vi "SV TDMS Write Even-Angle Channel Info.vi"(0 "tdms file":refnum<k34>, 1 "even-angle channel info":T6 {"channel info"."pregain" format="%.2f"; "channel info"."weighting filter" items=["Linear", "A-weighting", "B-weighting", "C-weighting", "ITU-R 468-4", "Dolby", "CCITT", "C-message", "Wb", "Wc", "Wd", "We", "Wf", "Wh", "Wj", "Wk", "Wm", "AES17 20 kHz lowpass", "AES17 40 kHz lowpass", "AES17 20 kHz highpass", "AES17 40 kHz highpass"]; "channel info"."dB reference" format="%^.1e"; "channel info"."engineering units" items=["custom..."=0, "V"=1, "A"=21, "C"=30, "pC"=31, "s"=32, "-"=29, "Pa"=2, "N"=20, "g"=3, "m/s^2"=4, "m/s"=5, "m"=6, "mm/s"=12, "mm"=13, "micron/s"=14, "micron"=15, "in/s^2"=7, "in/s"=8, "in"=9, "mil/s"=10, "mil"=11, "rad/s^2"=16, "rad/s"=17, "rad"=18, "deg/s^2"=26, "deg/s"=27, "deg"=28, "RPM"=22, "cycle/s^2"=23, "Hz"=24, "cycle"=25, "strain"=19]; "channel info"."sensor sensitivity" format="%#_5f"}, 5 "group name in":string, 7 "channel name in":string, 11 "error in":errorcluster) -> (4 "tdms file out":refnum<k34>, 6 "group name out":string, 8 "channel name out":string, 13 "function info":T5 {"function type" items=["Signal"=0, "Speed"=3, "Ratio"=6, "Count"=7, "-"=9, "Level"=10, "-"=19, "Octave Spectrum"=20, "-"=29, "FFT Auto Spectrum"=30, "FFT Cross Spectrum"=40, "Frequency Response"=50, "-"=59, "Event"=90]; "function subtype" items=["Unscaled binary"=0, "Scaled voltage"=1, "Scaled engineering units"=2, "-"=10, "Value"=19, "DC"=11, "AC"=12, "RMS^2"=13, "RMS"=14, "Peak"=15, "Peak to peak"=16, "-"=20, "1/1 octave"=21, "1/3 octave"=22, "1/6 octave"=23, "1/12 octave"=24, "1/24 octave"=25, "-"=30, "Density"=31, "Magnitude"=32, "Phase"=33, "Real"=34, "Imaginary"=35, "Complex"=345, "Coherence"=36, "-"=90, "Unknown"=99]; "X-domain" items=["Time (s)"=0, "Frequency-CB (Hz)"=1, "Frequency-CPB (Hz)"=1248, "Frequency-Arbitrary (Hz)"=2357, "Quefrency (s)"=2, "Revolutions (rev)"=3, "Order"=4, "Speed (RPM)"=11, "Speed (rad/s)"=21, "Index"=65535]}, 14 "unit info":T1, 15 "error out":errorcluster)   [LabVIEW 2017]
uses:
  <vilib>/addons/_NISVFA/_Shared subVIs/Controls/svc_Resampled Channel Info.ctl
  <vilib>/addons/_NISVFA/_Shared subVIs/Controls/svc_Channel Info.ctl
  <vilib>/addons/_NISVFA/_Shared subVIs/Controls/svc_Engineering Units Text Ring.ctl
  <vilib>/addons/_NISVFA/_Shared subVIs/Controls/svc_Weighting Filter Text Ring.ctl
  <vilib>/addons/_NISVFA/_Shared subVIs/Controls/NI Function Type.ctl
  <vilib>/addons/_NISVFA/_Shared subVIs/Controls/NI Function SubType.ctl
  <vilib>/addons/_NISVFA/_Shared subVIs/Controls/svc_X-Axis Units.ctl
  <vilib>/addons/_NISVFA/_Shared subVIs/Controls/svc_Unit Info.ctl
  <vilib>/addons/_NISVFA/_Shared subVIs/Controls/NI Channel Properties.ctl
  <vilib>/addons/_NISVFA/_Shared subVIs/Controls/SV Channel Properties.ctl
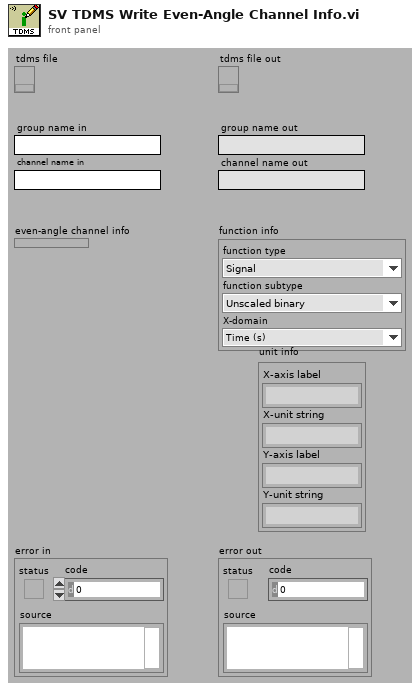
[diagram p1: front panel]
types:
  T1 = typedef "svc_Unit Info.ctl" = cluster{"X-axis label":string, "X-unit string":string, "Y-axis label":string, "Y-unit string":string}
  T2 = typedef "NI Function Type.ctl" = u16
  T3 = typedef "NI Function SubType.ctl" = u16
  T4 = typedef "svc_X-Axis Units.ctl" = u16
  T5 = cluster{"function type":T2, "function subtype":T3, "X-domain":T4}
  T6 = typedef "svc_Resampled Channel Info.ctl" = cluster{"channel name":string, "description":string, " channel info":T7}
  T7 = typedef "svc_Channel Info.ctl" = cluster{"sensor sensitivity":dbl, "engineering units":T8, "dB reference":dbl, "custom label":string, "weighting filter":T9, "pregain":dbl}
  T8 = typedef "svc_Engineering Units Text Ring.ctl" = u16
  T9 = typedef "svc_Weighting Filter Text Ring.ctl" = u16
  T10 = typedef "NI Channel Properties.ctl" = u16
  T11 = typedef "SV Channel Properties.ctl" = u16
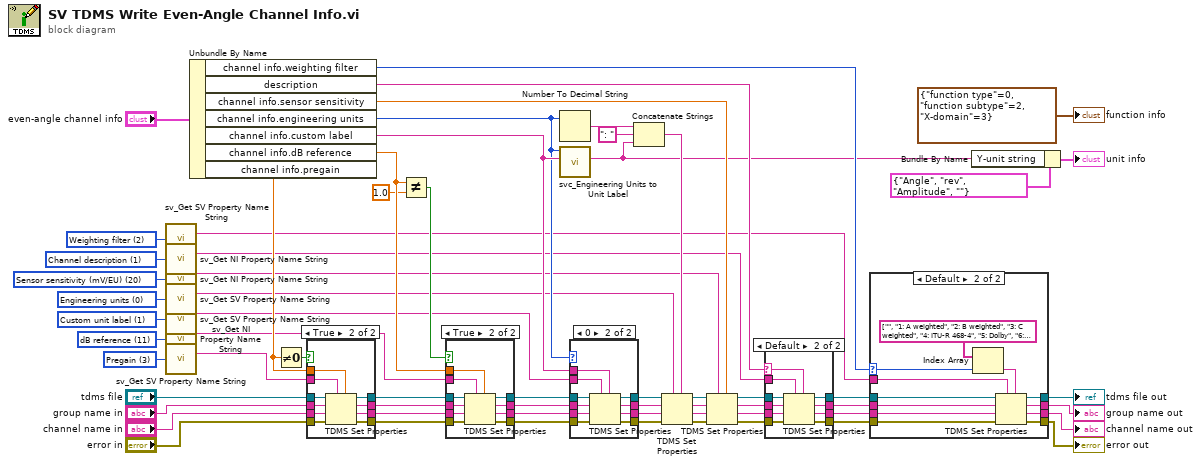
[diagram p0: block diagram]
diagram:
  w19 = T10 20 items=["Channel name", "Channel description", "Y-axis label", "Y-axis unit string", "X-axis label", "X-axis unit string", "x0", "dx", "Number of samples", "X channel", "Filter settled", "dB reference", "Window", "Window parameter", "Window size", "FFT size", "Peak units", "Spectrum type", "Magnitude scale", "Spectral density", "Sensor sensitivity (mV/EU)"] ("property")
  w17 = T10 11 items=["Channel name", "Channel description", "Y-axis label", "Y-axis unit string", "X-axis label", "X-axis unit string", "x0", "dx", "Number of samples", "X channel", "Filter settled", "dB reference", "Window", "Window parameter", "Window size", "FFT size", "Peak units", "Spectrum type", "Magnitude scale", "Spectral density"] ("property")
  w22 = T11 3 items=["Engineering units", "Custom unit label", "Weighting filter", "Pregain", "Octave standard", "Octave bandwidth", "Octave low band", "Octave high band", "Spectrum skewed"] ("SV property")
  w27 = T11 1 items=["Engineering units", "Custom unit label", "Weighting filter", "Pregain", "Octave standard", "Octave bandwidth", "Octave low band", "Octave high band", "Spectrum skewed"] ("SV property")
  w28 = T11 2 items=["Engineering units", "Custom unit label", "Weighting filter", "Pregain", "Octave standard", "Octave bandwidth", "Octave low band", "Octave high band", "Spectrum skewed"] ("SV property")
  w29 = T11 0 items=["Engineering units", "Custom unit label", "Weighting filter", "Pregain", "Octave standard", "Octave bandwidth", "Octave low band", "Octave high band", "Spectrum skewed"] ("SV property")
  w30 = T10 1 items=["Channel name", "Channel description", "Y-axis label", "Y-axis unit string", "X-axis label", "X-axis unit string", "x0", "dx", "Number of samples", "X channel", "Filter settled", "dB reference", "Window", "Window parameter", "Window size", "FFT size", "Peak units", "Spectrum type", "Magnitude scale", "Spectral density"] ("property")
  n1 = call <vilib>:"sv_Get SV Property Name String.vi"("property"=w28) -> ("TDMS property name"=w26:string)  [unwired: 13 in, 1 out]
  n2 = call <vilib>:"sv_Get NI Property Name String.vi"("property"=w30) -> ("TDMS property name"=w25:string)  [unwired: 13 in, 1 out]
  n3 = call <vilib>:"sv_Get NI Property Name String.vi"("property"=w19) -> ("TDMS property name"=w18:string)  [unwired: 13 in, 1 out]
  n4 = call <vilib>:"sv_Get SV Property Name String.vi"("property"=w29) -> ("TDMS property name"=w24:string)  [unwired: 13 in, 1 out]
  n5 = call <vilib>:"sv_Get SV Property Name String.vi"("property"=w27) -> ("TDMS property name"=w23:string)  [unwired: 13 in, 1 out]
  n6 = call <vilib>:"sv_Get NI Property Name String.vi"("property"=w17) -> ("TDMS property name"=w20:string)  [unwired: 13 in, 1 out]
  n7 = call <vilib>:"sv_Get SV Property Name String.vi"("property"=w22) -> ("TDMS property name"=w21:string)  [unwired: 13 in, 1 out]
  n8 = Unbundle By Name("even-angle channel info") -> ("channel info.weighting filter"=w42:T9, "description"=w43:string, "channel info.sensor sensitivity"=w60:dbl, "channel info.engineering units"=w49:T8, "channel info.custom label"=w50:string, "channel info.dB reference"=w48:dbl, "channel info.pregain"=w44:dbl)
  n9 = Not Equal To 0?(x=w44) -> (x != 0?=w45:bool)
  n10 = case shown="True" w45 {
    tunnel: [w65 w78] -> w32
    tunnel: [w66 w77] -> w33
    tunnel: [w67 w76] -> w34
    tunnel: [w68 w75] -> w35
    tunnel: w44 -> [_ w69]
    tunnel: w21 -> [_ w74]
    tunnel: "tdms file" -> [w68 w73]
    tunnel: "group name in" -> [w67 w72]
    tunnel: "channel name in" -> [w66 w71]
    tunnel: "error in" -> [w65 w70]
    frame False {
    }
    frame True {
      n11 = TDMS Set Properties(5:w69, 7:w74, 8:w70, 9:w71, 10:w72, 11:w73) -> (0:w78:errorcluster, 1:w77:string, 2:w76:string, 3:w75:refnum<k34>)
    }
  }
  n12 = Not Equal?(x=w48, y=1.0) -> (x != y?=w47:bool)
  n13 = case shown="True" w47 {
    tunnel: w32 -> [w79 w92]
    tunnel: w33 -> [w80 w91]
    tunnel: w34 -> [w81 w90]
    tunnel: w35 -> [w82 w89]
    tunnel: [w79 w88] -> w36
    tunnel: [w80 w87] -> w37
    tunnel: [w81 w86] -> w38
    tunnel: [w82 w85] -> w39
    tunnel: w48 -> [_ w84]
    tunnel: w20 -> [_ w83]
    frame False {
    }
    frame True {
      n14 = TDMS Set Properties(5:w84, 7:w83, 8:w92, 9:w91, 10:w90, 11:w89) -> (0:w88:errorcluster, 1:w87:string, 2:w86:string, 3:w85:refnum<k34>)
    }
  }
  n15 = Number To Decimal String(number=w49) -> (decimal integer string=w41:string)  [unwired: 1 in]
  n16 = call <vilib>:"svc_Engineering Units to Unit Label.vi"("custom label"=w50, "engineering units"=w49) -> ("unit label"=w14:string)  [unwired: 8 in, 1 out]
  n17 = case shown="0" w49 {
    tunnel: w36 -> [w93 w106]
    tunnel: w37 -> [w94 w105]
    tunnel: w38 -> [w95 w104]
    tunnel: w39 -> [w96 w103]
    tunnel: [w93 w102] -> w10
    tunnel: [w94 w101] -> w11
    tunnel: [w95 w100] -> w12
    tunnel: [w96 w99] -> w13
    tunnel: w23 -> [_ w98]
    tunnel: w50 -> [_ w97]
    frame Default {
    }
    frame 0 {
      n18 = TDMS Set Properties(5:w97, 7:w98, 8:w106, 9:w105, 10:w104, 11:w103) -> (0:w102:errorcluster, 1:w101:string, 2:w100:string, 3:w99:refnum<k34>)
    }
  }
  n19 = Concatenate Strings(w41, ": " ("string"), w14) -> (w51:string)
  n20 = TDMS Set Properties(5:w51, 7:w24, 8:w10, 9:w11, 10:w12, 11:w13) -> (0:w52:errorcluster, 1:w53:string, 2:w54:string, 3:w55:refnum<k34>)
  n21 = TDMS Set Properties(5:w60, 7:w18, 8:w52, 9:w53, 10:w54, 11:w55) -> (0:w59:errorcluster, 1:w58:string, 2:w57:string, 3:w56:refnum<k34>)
  n22 = case shown="Default" w43 {
    selector: w43 -> [_ w111]
    tunnel: [w107 w120] -> w2
    tunnel: [w108 w119] -> w3
    tunnel: [w109 w118] -> w4
    tunnel: [w110 w117] -> w5
    tunnel: w25 -> [_ w116]
    tunnel: w56 -> [w110 w115]
    tunnel: w57 -> [w109 w114]
    tunnel: w58 -> [w108 w113]
    tunnel: w59 -> [w107 w112]
    frame "" {
    }
    frame Default {
      n23 = TDMS Set Properties(5:w111, 7:w116, 8:w112, 9:w113, 10:w114, 11:w115) -> (0:w120:errorcluster, 1:w119:string, 2:w118:string, 3:w117:refnum<k34>)
    }
  }
  n24 = case shown="Default" w42 {
    selector: w42 -> [_ w127]
    tunnel: w2 -> [w121 w136]
    tunnel: w3 -> [w122 w135]
    tunnel: w4 -> [w123 w134]
    tunnel: w5 -> [w124 w133]
    tunnel: [w124 w132] -> w61
    tunnel: [w123 w131] -> w62
    tunnel: [w122 w130] -> w63
    tunnel: [w121 w129] -> w64
    tunnel: w26 -> [_ w128]
    frame 0 {
    }
    frame Default {
      n25 = Index Array(array=string[] ["", "1: A weighted", "2: B weighted", "3: C weighted", "4: ITU-R 468-4", "5: Dolby", "6: CCITT", "7: C-message", "8: Wb", "9: Wc", "10: Wd", "11: We", "12: Wf", "13: Wh", "14: Wj", "15: Wk", "16: Wm"] ("transposed array"), index=w127) -> (element=w125:string)
      n26 = TDMS Set Properties(5:w125, 7:w128, 8:w136, 9:w135, 10:w134, 11:w133) -> (0:w129:errorcluster, 1:w130:string, 2:w131:string, 3:w132:refnum<k34>)
    }
  }
  "error out" <- w64
  "channel name out" <- w63
  "group name out" <- w62
  "tdms file out" <- w61
  n27 = Bundle By Name(cluster=T1 {"X-axis label"="Angle", "X-unit string"="rev", "Y-axis label"="Amplitude", "Y-unit string"=""} ("unit info 2"), "Y-unit string"=w14) -> (→"unit info":T1)
  "function info" <- T5 {"function type"=0, "function subtype"=2, "X-domain"=3} ("function info")
